vi "find readout time.vi"(8 "error in (no error)":errorcluster, 11 "Simulated_CCD_Camera in":refnum<class "Simulated Camera.lvclass">) -> (0 "error out":errorcluster, 3 "Simulated_CCD_Camera out":refnum<class "Simulated Camera.lvclass">)   [LabVIEW 2018, in "Simulated Camera.lvclass"]
doc: "Find the readout time as a function of the operation mode of the CCD.\n\nThis value is used to determine the minimum exposure time allowed by ACS, that is the readout time plus 10 % of this value. This procedure is related to the functioning of the frame transfer mode of the CCD and it prevents the misuse of the exposure time."
uses:
  Simulated Camera.lvclass
  Simulated Camera.lvclass/Simulated Camera.ctl
  <vilib>/Utility/file.llb/Read Delimited Spreadsheet (DBL).vi
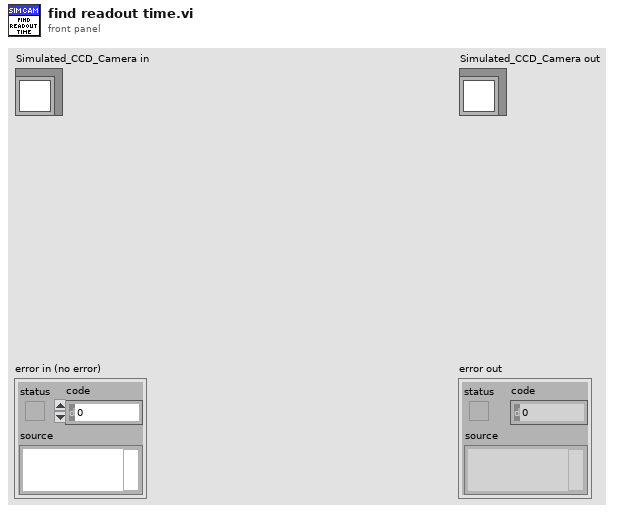
[diagram p1: front panel]
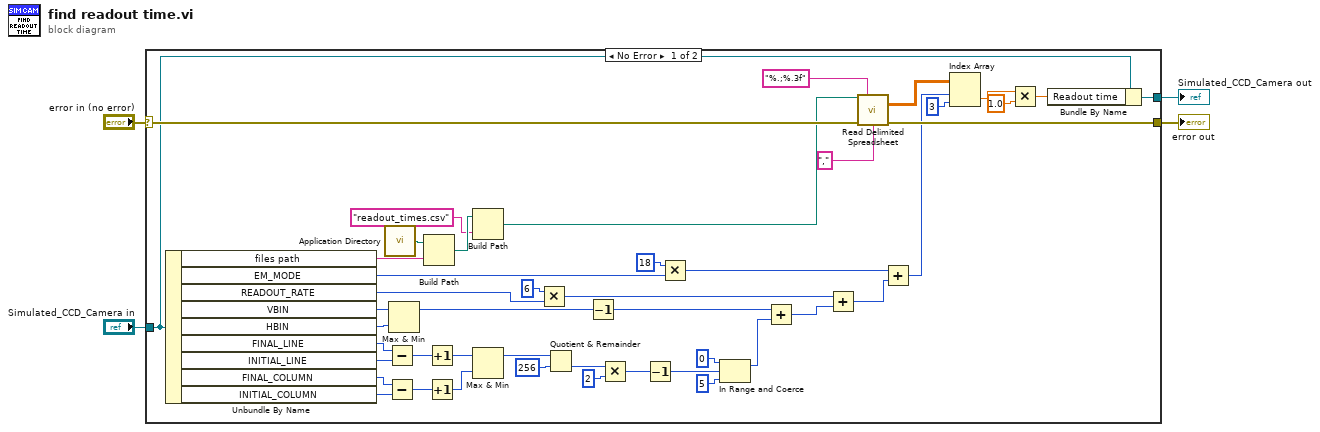
[diagram p0: block diagram]
diagram:
  n1 = case shown="No Error" "error in (no error)" {
    selector: "error in (no error)" -> [w50 w52]
    tunnel: [w49 w52] -> w3
    tunnel: [w11 w51] -> w1
    tunnel: "Simulated_CCD_Camera in" -> [w12 w51]
    frame No Error {
      n2 = Unbundle By Name(w12) -> ("files path"=w5:string, "EM_MODE"=w28:u16, "READOUT_RATE"=w32:u16, "VBIN"=w36:u16, "HBIN"=w35:u16, "FINAL_LINE"=w44:u16, "INITIAL_LINE"=w43:u16, "FINAL_COLUMN"=w42:u16, "INITIAL_COLUMN"=w41:u16)
      n3 = call <vilib>:"Application Directory.vi"() -> ("Application Directory"=w47:path)
      n4 = Subtract(x=w44, y=w43) -> (x-y=w46:u16)
      n5 = Subtract(x=w42, y=w41) -> (x-y=w45:u16)
      n6 = Max & Min(x=w36, y=w35) -> (max(x,y)=w34:u16)  [unwired: 1 out]
      n7 = Build Path(base path=w47, name or relative path=w5) -> (appended path=w9:path)
      n8 = Increment(x=w46) -> (x+1=w40:u16)
      n9 = Increment(x=w45) -> (x+1=w39:u16)
      n10 = Build Path(base path=w9, name or relative path="readout_times.csv") -> (appended path=w8:path)
      n11 = Max & Min(x=w40, y=w39) -> (max(x,y)=w37:u16)  [unwired: 1 out]
      n12 = Multiply(x=u16 6, y=w32) -> (x*y=w29:u16)
      n13 = Quotient & Remainder(x=w37, y=u16 256) -> (floor(x/y)=w19:u16)  [unwired: 1 out]
      n14 = Decrement(x=w34) -> (x-1=w33:u16)
      n15 = Multiply(x=w19, y=u16 2 ("x")) -> (x*y=w20:u16)
      n16 = Decrement(x=w20) -> (x-1=w18:u16)
      n17 = Multiply(x=u16 18, y=w28) -> (x*y=w25:u16)
      n18 = In Range and Coerce(upper limit=u16 0, x=w18, lower limit=u16 5 ("upper limit")) -> (coerced(x)=w15:u16)  [unwired: 1 out]
      n19 = Add(x=w33, y=w15) -> (x+y=w30:u16)
      n20 = Add(x=w29, y=w30) -> (x+y=w26:u16)
      n21 = call-poly <vilib>:"Read Delimited Spreadsheet.vi"("file path (dialog if empty)"=w8, "format (%.3f)"="%.;%.3f", "error in (no error)"=w50, "delimiter (\\t)"="," ("delimiter (\\t)")) -> ("all rows"=w24:dbl[][], "error out"=w49:errorcluster)  [unwired: 6 in, 4 out]
      n22 = Add(x=w25, y=w26) -> (x+y=w22:u16)
      n23 = Index Array(array=w24, index (row)=w22, index (col)=3 ("disabled index (col)")) -> (element=w14:dbl)
      n24 = Multiply(x=w14, y=1.0) -> (x*y=w10:dbl)
      n25 = Bundle By Name(cluster=w12, "Readout time"=w10) -> (w11:refnum<class "Simulated Camera.lvclass">)
    }
    frame Error {
    }
  }
  "error out" <- w3
  "Simulated_CCD_Camera out" <- w1
